vi "ConfigWriter.vi"(0 "Path":path, 1 "Mode":bool, 2 "Syringe Volume":i32=3 min=0 max=100 step=1, 4 "Withdraw \nVolume unit":u16(ring) items=["µL", "nL", "mL"], 5 "error in (no error)":errorcluster, 7 "Withdraw rate":dbl=2.0, 8 "Withdraw Rate \nUnits":u32(ring)=3 items=["ml/hr", "ml/min", "ul/hr", "ul/min", "ul/sec", "nl/sec"], 10 "Withdraw \nVolume":i32=100, 11 "Syringe Diameter (mm)":dbl=4.86 min=0.01 max=49.99 step=0.01 format="%.2g", 12 "Infusion rate":dbl=2.0 min=0.0 max=999.0 step=0.1, 13 "Infusion Rate Units":u32(ring)=3 items=["ml/hr", "ml/min", "ul/hr", "ul/min", "ul/sec", "nl/sec"], 14 "Infusion volume":i32=100, 15 "Infusion volume unit":u16(ring) items=["µL", "nL", "mL"], 17 "Current Force":i32=30 min=0 max=100 step=1, 18 "Syringe Volume Unit":u16(ring)=2 items=["µL", "nL", "mL"]) -> (19 "error out":errorcluster)   [LabVIEW 2016]
uses:
  <vilib>/Utility/config.llb/Write Key (Double).vi
  <vilib>/Utility/config.llb/Write Key (U32).vi
  <vilib>/Utility/config.llb/Write Key (I32).vi
  <vilib>/Utility/config.llb/Write Key (String).vi
  <vilib>/Utility/config.llb/NI_LVConfig.lvlib
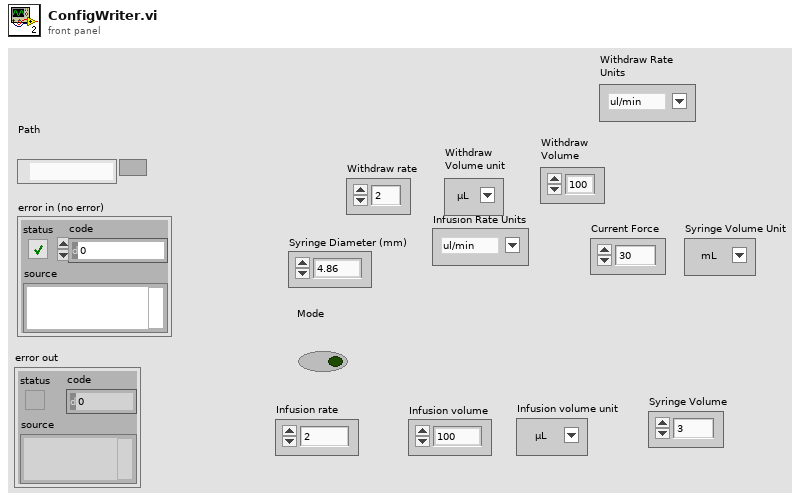
[diagram p1: front panel]
types:
  T1 = typedef "NI_LVConfig.lvlib/Config Data RefNum.ctl" = refnum<k1>
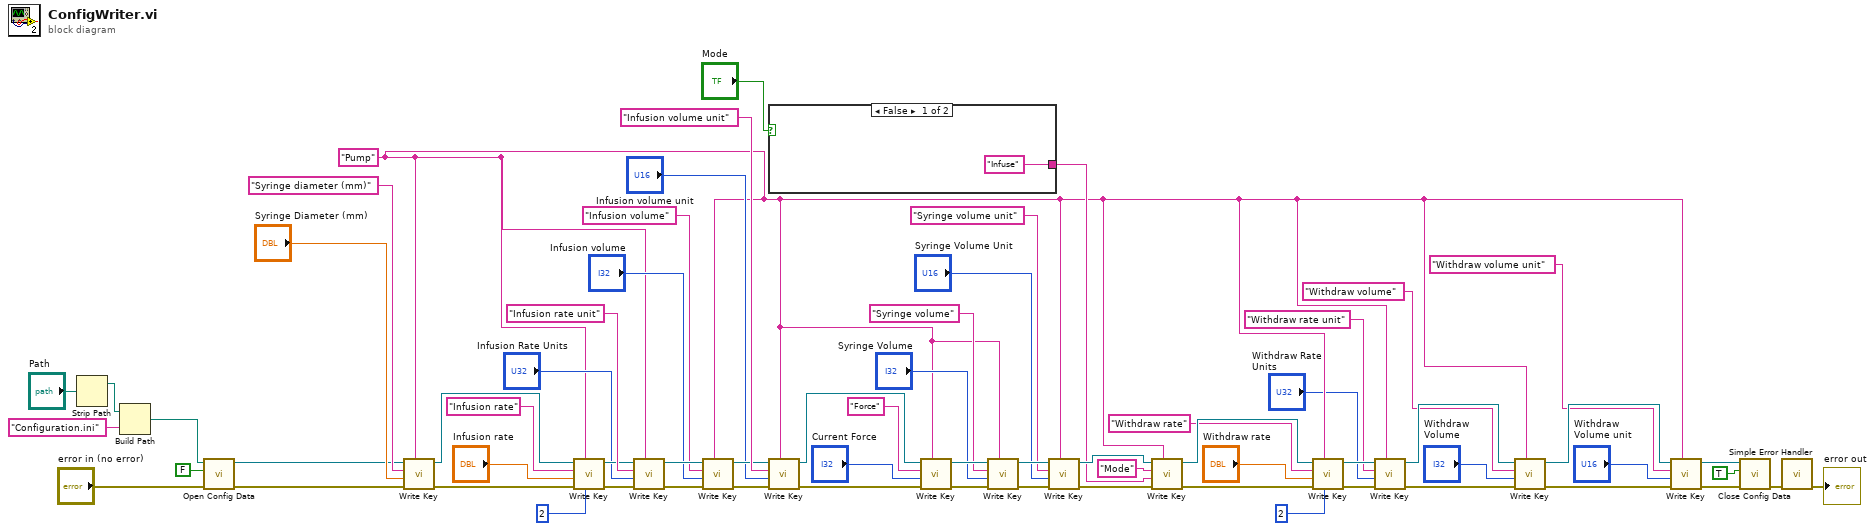
[diagram p0: block diagram]
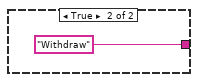
[diagram p2: hidden frame]
diagram:
  w13 = "Pump" ("section")
  n1 = Strip Path(path="Path") -> (stripped path=w51:path)  [unwired: 1 out]
  n2 = Build Path(base path=w51, name or relative path="Configuration.ini") -> (appended path=w49:path)
  n3 = call <vilib>:"Open Config Data.vi"("error in (no error)"="error in (no error)", "create file if necessary (T)"=FALSE, "configuration file path"=w49) -> ("error out"=w3:errorcluster, "refnum"=w4:T1)  [unwired: 6 in, 1 out]
  n4 = call-poly <vilib>:"Write Key.vi"("section"=w13, "error in (no error)"=w3, "value"="Syringe Diameter (mm)", "key"="Syringe diameter (mm)", "refnum"=w4) -> ("error out"=w62:errorcluster, "refnum out"=w53:T1)  [unwired: 4 in, 1 out]
  n5 = call-poly <vilib>:"Write Key.vi"("precision (6)"=i16 2, "section"=w13, "error in (no error)"=w62, "value"="Infusion rate", "key"="Infusion rate", "refnum"=w53) -> ("error out"=w63:errorcluster, "refnum out"=w54:T1)  [unwired: 3 in, 1 out]
  n6 = call-poly <vilib>:"Write Key.vi"("section"=w13, "error in (no error)"=w63, "value"="Infusion Rate Units", "key"="Infusion rate unit", "refnum"=w54) -> ("error out"=w64:errorcluster, "refnum out"=w55:T1)  [unwired: 4 in, 1 out]
  n7 = call-poly <vilib>:"Write Key.vi"("section"=w13, "error in (no error)"=w64, "value"="Infusion volume", "key"="Infusion volume", "refnum"=w55) -> ("error out"=w65:errorcluster, "refnum out"=w56:T1)  [unwired: 4 in, 1 out]
  n8 = case shown="False" "Mode" {
    tunnel: ["Infuse" "Withdraw"] -> w24
    frame False {
    }
    frame True {
    }
  }
  n9 = call-poly <vilib>:"Write Key.vi"("section"=w13, "error in (no error)"=w65, "value"="Infusion volume unit", "key"="Infusion volume unit", "refnum"=w56) -> ("error out"=w47:errorcluster, "refnum out"=w66:T1)  [unwired: 4 in, 1 out]
  n10 = call-poly <vilib>:"Write Key.vi"("section"=w13, "error in (no error)"=w47, "value"="Current Force", "key"="Force", "refnum"=w66) -> ("error out"=w34:errorcluster, "refnum out"=w36:T1)  [unwired: 4 in, 1 out]
  n11 = call-poly <vilib>:"Write Key.vi"("section"=w13, "error in (no error)"=w34, "value"="Syringe Volume", "key"="Syringe volume", "refnum"=w36) -> ("error out"=w33:errorcluster, "refnum out"=w35:T1)  [unwired: 4 in, 1 out]
  n12 = call-poly <vilib>:"Write Key.vi"("section"=w13, "error in (no error)"=w33, "value"="Syringe Volume Unit", "key"="Syringe volume unit", "refnum"=w35) -> ("error out"=w27:errorcluster, "refnum out"=w28:T1)  [unwired: 4 in, 1 out]
  n13 = call-poly <vilib>:"Write Key.vi"("section"=w13, "error in (no error)"=w27, "value"=w24, "key"="Mode", "refnum"=w28) -> ("error out"=w20:errorcluster, "refnum out"=w21:T1)  [unwired: 4 in, 1 out]
  n14 = call-poly <vilib>:"Write Key.vi"("precision (6)"=i16 2, "section"=w13, "error in (no error)"=w20, "value"="Withdraw rate", "key"="Withdraw rate", "refnum"=w21) -> ("error out"=w22:errorcluster, "refnum out"=w23:T1)  [unwired: 3 in, 1 out]
  n15 = call-poly <vilib>:"Write Key.vi"("section"=w13, "error in (no error)"=w22, "value"="Withdraw Rate \nUnits", "key"="Withdraw rate unit", "refnum"=w23) -> ("error out"=w16:errorcluster, "refnum out"=w17:T1)  [unwired: 4 in, 1 out]
  n16 = call-poly <vilib>:"Write Key.vi"("section"=w13, "error in (no error)"=w16, "value"="Withdraw \nVolume", "key"="Withdraw volume", "refnum"=w17) -> ("error out"=w18:errorcluster, "refnum out"=w19:T1)  [unwired: 4 in, 1 out]
  n17 = call-poly <vilib>:"Write Key.vi"("section"=w13, "error in (no error)"=w18, "value"="Withdraw \nVolume unit", "key"="Withdraw volume unit", "refnum"=w19) -> ("error out"=w14:errorcluster, "refnum out"=w15:T1)  [unwired: 4 in, 1 out]
  n18 = call <vilib>:"Close Config Data.vi"("error in (no error)"=w14, "write file if changed (T)"=TRUE, "refnum"=w15) -> ("error out"=w44:errorcluster)  [unwired: 7 in, 1 out]
  n19 = call <vilib>:"Simple Error Handler.vi"("error in (no error)"=w44) -> ("error out"=→"error out":errorcluster)  [unwired: 4 in, 4 out]
